vi "vipbBuild.vi"() -> (0 "error out":errorcluster)   [LabVIEW 2014, in "lv-cli-steps.lvlib"]
uses:
  lv-cli-steps.lvlib
  <vilib>/Utility/error.llb/DialogType.ctl
  <vilib>/Wiresmith Technology/LabVIEW CLI/CLI Class/CLI.lvclass
  <vilib>/JKI/VIPM API/VIPM API_vipm_api.lvlib
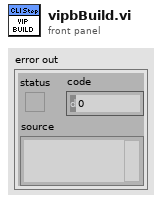
[diagram p1: front panel]
types:
  T1 = typedef "DialogType.ctl" = u16
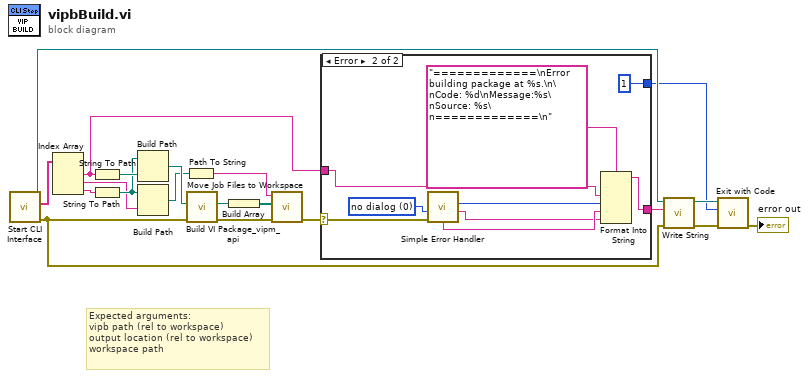
[diagram p0: block diagram]
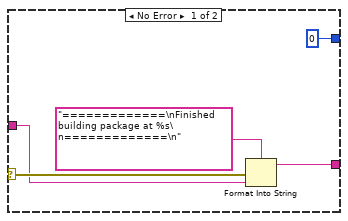
[diagram p2: hidden frame]
diagram:
  # "Expected arguments:\nvipb path (rel to workspace)\noutput location (rel to workspace)\nworkspace path"
  n1 = call <vilib>:"Start CLI Interface.vi"() -> ("error out"=w8:errorcluster, "Custom Parameters"=w20:string[], "CLI out"=w18:refnum<class "CLI.lvclass">)  [unwired: 9 in]
  n2 = Index Array(array=w20) -> (element #1=w6:string, element #2=w3:string, element #3=w5:string)  [unwired: 3 in]
  n3 = String To Path(string=w6) -> (path=w14:path)
  n4 = String To Path(string=w5) -> (path=w4:path)
  n5 = Build Path(base path=w4, name or relative path=w14) -> (appended path=w7:path)
  n6 = Build Path(base path=w4, name or relative path=w3) -> (appended path=w1:path)
  n7 = Path To String(path=w1) -> (string=w2:string)
  n8 = call <vilib>:"Build VI Package_vipm_api.vi"("error in (no error)"=w8, "Path to VIPB File"=w7) -> ("error out"=w9:errorcluster, "Build Output"=w11:path)  [unwired: 8 in]
  n9 = Build Array(w11) -> (w10:path[])
  n10 = call "Move Job Files to Workspace.vi"("error in (no error)"=w9, "Generated Files"=w10, "Workspace Path"=w2) -> ("error out"=w13:errorcluster)  [unwired: 8 in]
  n11 = case shown="Error" w13 {
    selector: w13 -> [w24 w33]
    tunnel: w6 -> [w23 w29]
    tunnel: [w22 w34] -> w19
    tunnel: [0 ("Exit Code (0)") 1 ("Exit Code (0)")] -> w15
    frame No Error {
      n12 = Format Into String(format string="=============\nFinished building package at %s\n=============\n", error in=w24, w23) -> (resulting string=w22:string)  [unwired: 1 in, 1 out]
    }
    frame Error {
      w32 = T1 0 items=["no dialog", "OK message", "continue or stop message", "OK message + warnings", "continue/stop + warnings"] ("type of dialog (OK msg:1)")
      n13 = call <vilib>:"Simple Error Handler.vi"("type of dialog (OK msg:1)"=w32, "error in (no error)"=w33) -> ("code out"=w26:i32, "source out"=w27:string, "message"=w28:string)  [unwired: 3 in, 2 out]
      n14 = Format Into String(format string="=============\nError building package at %s.\n\nCode: %d\nMessage:%s\nSource: %s\n=============\n", w29, w26, w28, w27) -> (resulting string=w34:string)  [unwired: 2 in, 1 out]
    }
  }
  n15 = call <vilib>:"Write String.vi"("error in (no error)"=w8, "Text to Write"=w19, "CLI in"=w18) -> ("error out"=w17:errorcluster, "CLI out"=w16:refnum<class "CLI.lvclass">)  [unwired: 7 in]
  n16 = call <vilib>:"Exit with Code.vi"("error in (no error)"=w17, "Exit Code (0)"=w15, "CLI in"=w16) -> ("error out"=→"error out":errorcluster)  [unwired: 8 in]
